vi "C Parent.vi"() -> ()   [LabVIEW 2016]
panel:
  out "Units":string
  out "th, Theta":dbl
  in  "x, Original Value":dbl
  in  "Output in Degrees or Radians?":string(combo)
  in  "Inverse Trig Function":string(combo)
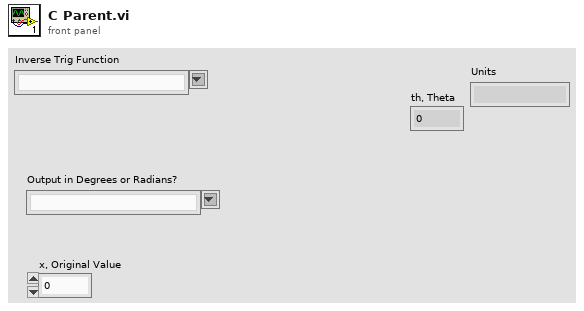
[diagram p1: front panel]
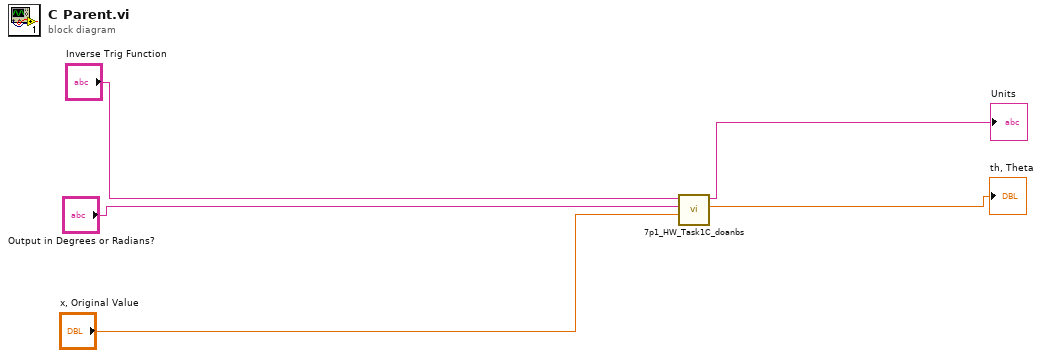
[diagram p0: block diagram]
diagram:
  n1 = call "7p1_HW_Task1C_doanbs.vi"("x, Original Value"="x, Original Value", "Output in Degrees or Radians?"="Output in Degrees or Radians?", "Inverse Trig Function"="Inverse Trig Function") -> ("th, Theta"=→"th, Theta":dbl, "Units"=→"Units":string)  [unwired: 7 in]
